vi "UTIL_Timer.vi"(8 "Auto Reset":bool=TRUE, 9 "Reset":bool, 10 "Time (sec)":dbl=3.0, 11 "Start":bool) -> (0 "Timed Out":bool, 1 "Running":bool, 2 "Numeric 2":dbl, 3 "Numeric":dbl, 4 "TO Trig":bool)   [LabVIEW 2024]
doc: "Uses the second timer to determind when Time (sec) have passed when Start is TRUE. The actual time passes is captured in Lap (sec) \nAutoReset is enabled by default. When enabled, at time out, the values is captured, and the TimeOut set to TRUE for one loop then both are RESET. When not enabled, then a RESET command or another START command are requied to reset both the value and TimeOut Flag.\n\n(The functionality could be expanded to measure elapse time on Mark.)"
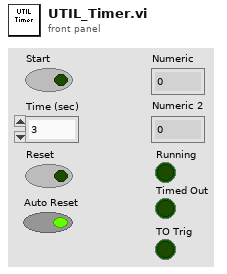
[diagram p1: front panel]
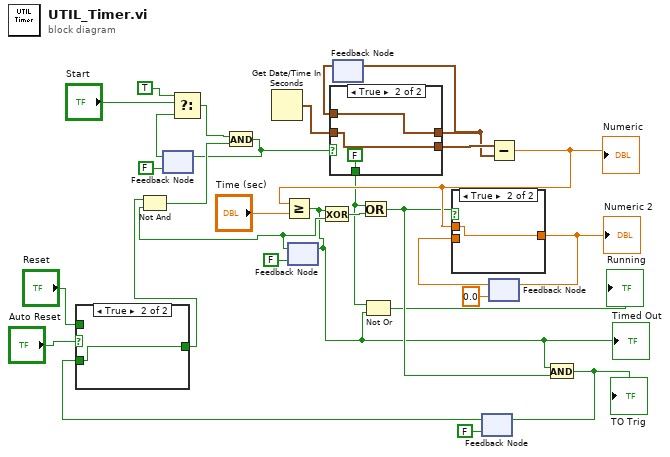
[diagram p0: block diagram]
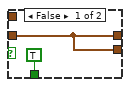
[diagram p4: hidden frame]
diagram:
  n1 = feedback #1(FALSE) -> (w16:bool)
  n2 = Select(t=TRUE, s="Start", f=w16) -> (s? t:f=w14:bool)
  n3 = Get Date/Time In Seconds() -> (seconds since 1Jan1904=w19:timestamp)
  n4 = feedback #2(FALSE) -> (w13:bool)
  n5 = feedback #3() -> (w20:timestamp)  [unwired: 1 in]
  n6 = feedback #4(FALSE) -> (w5:bool)
  n7 = case shown="True" "Auto Reset" {
    tunnel: "Reset" -> [w30 _]
    tunnel: [w30 w31] -> w8
    tunnel: w5 -> [_ w31]
    frame False {
    }
    frame True {
    }
  }
  n8 = Not And(1:w13, 2:w8) -> (0:w12:bool)
  n9 = And(x=w14, y=w12) -> (x .and. y?=w11:bool)
  n10 = feedback-in #1(w11) -> ()
  n11 = case shown="True" w11 {
    tunnel: w19 -> [w33 w35]
    tunnel: [w33 w36] -> w21
    tunnel: w20 -> [_ w36]
    tunnel: [w33 w35] -> w22
    tunnel: [TRUE FALSE] -> w3
    frame False {
    }
    frame True {
    }
  }
  n12 = feedback-in #3(w21) -> ()
  n13 = Subtract(x=w22, y=w21) -> (x-y=w27:dbl)
  "Numeric" <- w27
  n14 = Greater Or Equal?(x=w27, y="Time (sec)") -> (x >= y?=w1:bool)
  "Timed Out" <- w1
  n15 = feedback-in #2(w1) -> ()
  n16 = Exclusive Or(1:w13, 2:w1) -> (0:w28:bool)
  n17 = Or(x=w3, y=w28) -> (x .or. y?=w10:bool)
  n18 = Not Or(1:w1, 2:w3) -> (0:→"Running":bool)
  n19 = feedback #5(0.0) -> (w24:dbl)
  n20 = case shown="True" w10 {
    tunnel: [w37 w38] -> w23
    tunnel: w24 -> [w37 _]
    tunnel: w27 -> [_ w38]
    frame False {
    }
    frame True {
    }
  }
  "Numeric 2" <- w23
  n21 = feedback-in #5(w23) -> ()
  n22 = And(x=w1, y=w10) -> (x .and. y?=w7:bool)
  "TO Trig" <- w7
  n23 = feedback-in #4(w7) -> ()
